vi "Holo Position SLM.vi"(5 "y":string, 9 "x":string) -> (6 "x-y":dbl, 10 "x-y 2":dbl)   [LabVIEW 2014]
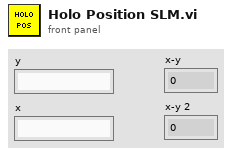
[diagram p1: front panel]
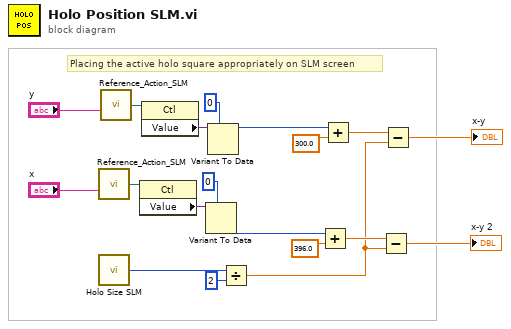
[diagram p0: block diagram]
diagram:
  # "Placing the active holo square appropriately on SLM screen"
  n1 = call "Reference_Action_SLM.vi"("Control Name"="x") -> ("Ref OUT"=w12:refnum<vi>)  [unwired: 12 in, 2 out]
  n2 = call "Holo Size SLM.vi"() -> ("data"=w13:i32)  [unwired: 15 in]
  n3 = call "Reference_Action_SLM.vi"("Control Name"="y") -> ("Ref OUT"=w9:refnum<vi>)  [unwired: 12 in, 2 out]
  n4 = property class="Ctl"(reference=w12) -> ("Value"=w11:variant)  [unwired: 1 in, 2 out]
  n5 = property class="Ctl"(reference=w9) -> ("Value"=w8:variant)  [unwired: 1 in, 2 out]
  n6 = Variant To Data(type=0, Variant=w11) -> (data=w5:i32)  [unwired: 1 in, 1 out]
  n7 = Variant To Data(type=0, Variant=w8) -> (data=w6:i32)  [unwired: 1 in, 1 out]
  n8 = Divide(x=w13, y=2) -> (x/y=w16:dbl)
  n9 = Add(x=w5, y=396.0 ("x")) -> (x+y=w18:dbl)
  n10 = Add(x=w6, y=300.0 ("x")) -> (x+y=w17:dbl)
  n11 = Subtract(x=w18, y=w16) -> (x-y=→"x-y 2":dbl)
  n12 = Subtract(x=w17, y=w16) -> (x-y=→"x-y":dbl)
